vi "Read Access.vi"(11 "WPL Comm in":refnum<class "WPL Comm.lvclass">) -> (2 "Access":T1, 3 "WPL Comm out":refnum<class "WPL Comm.lvclass">)   [LabVIEW 2020, in "Internal Comm Classes.lvlib" / "WPL Comm.lvclass"]
uses:
  WPL Comm.lvclass
  Access mode.ctl
  WPL Comm.lvclass/WPL Comm.ctl
  NI_VS Custom Device Waveform API.lvlib
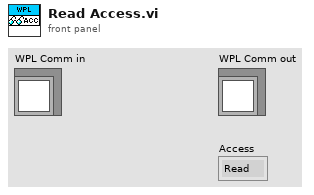
[diagram p1: front panel]
types:
  T1 = typedef "NI_VS Custom Device Waveform API.lvlib/Access mode.ctl" = enum16{"Read", "Write"}
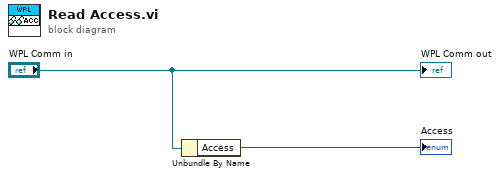
[diagram p0: block diagram]
diagram:
  n1 = Unbundle By Name("WPL Comm in") -> ("Access"=→"Access":T1)
  "WPL Comm out" <- "WPL Comm in"
